vi "Player Info.vi"(8 "Victory Speech":string="The Lone Wolf Runs Alone", 9 "Name":string="Lone Wolf", 11 "Lone Wolf in":refnum<class "Lone Wolf.lvclass">) -> (3 "Lone Wolf out":refnum<class "Lone Wolf.lvclass">)   [LabVIEW 2015, in "Lone Wolf.lvclass"]
uses:
  Lone Wolf.lvclass
  Square/Square.lvclass
panel:
  # "Set default values for these two string controls"
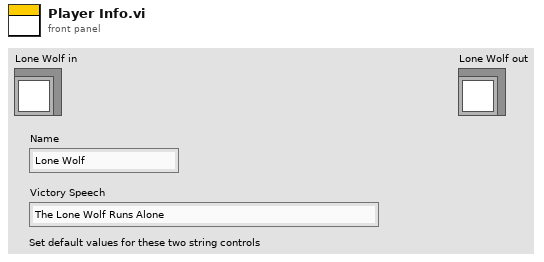
[diagram p1: front panel]
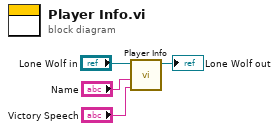
[diagram p0: block diagram]
diagram:
  n1 = call-parent "Player Info.vi"("Victory Speech"="Victory Speech", "Name"="Name", "Square in"="Lone Wolf in") -> ("Square out"=→"Lone Wolf out":refnum<class "Lone Wolf.lvclass">)  [unwired: 8 in]
